vi "Set ClassID.vi"(8 "error in (no error)":errorcluster caption="错误输入（无错误）", 10 "ClassID":u32, 11 "Generic输入":refnum<class "Generic.lvclass">) -> (0 "error out":errorcluster caption="错误输出", 3 "Generic输出":refnum<class "Generic.lvclass">)   [LabVIEW 2013, in "Hierarchy Framework.lvlib" / "Generic.lvclass"]
uses:
  Generic.lvclass
  Generic.lvclass/Generic.ctl
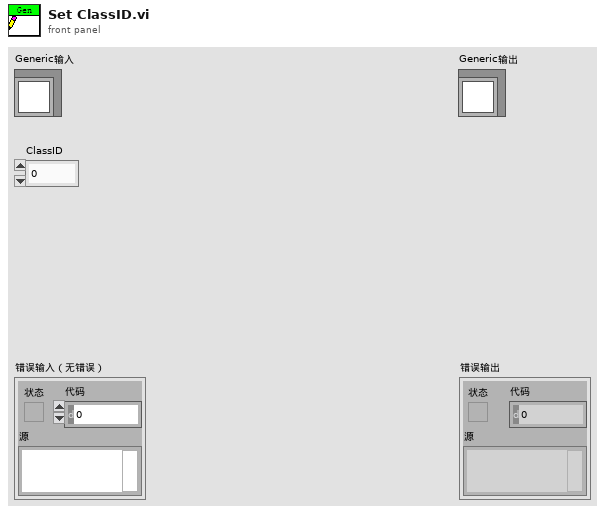
[diagram p1: front panel]
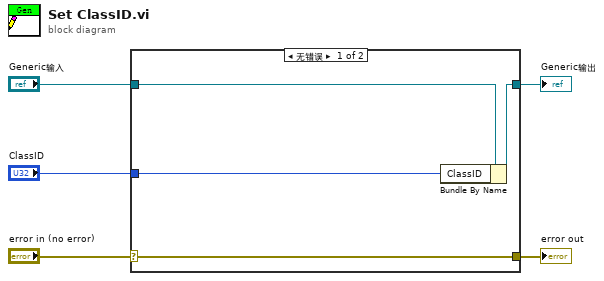
[diagram p0: block diagram]
diagram:
  n1 = case shown="无错误" "error in (no error)" {
    selector: "error in (no error)" -> [w9 w10]
    tunnel: [w9 w10] -> w4
    tunnel: [w7 w11] -> w2
    tunnel: "Generic输入" -> [w8 w11]
    tunnel: "ClassID" -> [w6 _]
    frame No Error {
      n2 = Bundle By Name(cluster=w8, "ClassID"=w6) -> (w7:refnum<class "Generic.lvclass">)
    }
    frame Error {
    }
  }
  "error out" <- w4
  "Generic输出" <- w2
